vi "Send Update Data Buffer.vi"(6 "gain":dbl, 7 "Message Priority (Normal)":T2=enum."Normal", 8 "error in (no error)":errorcluster, 9 "dt":dbl, 10 "Data Buffer":T1, 11 "Message Enqueuer":refnum<class "Message Enqueuer.lvclass">) -> (0 "error out":errorcluster, 3 "Message Enqueuer out":refnum<class "Message Enqueuer.lvclass">)   [LabVIEW 2020, in "Calculation Worker.lvlib" / "Update Data Buffer Msg.lvclass"]
doc: "This VI sends the message to an actor."
uses:
  Update Data Buffer Msg.lvclass
  <vilib>/ActorFramework/Message Enqueuer/Message Enqueuer.lvclass
  <vilib>/ActorFramework/Message Enqueuer/Message Priority.ctl
  GPU FFT Calculator/GPU FFT Calculator/Data Source Buffer.ctl
  C:/Program Files/National Instruments/LabVIEW 2026/vi.lib/ActorFramework/Message/Message.lvclass
  Update Data Buffer Msg.lvclass/Update Data Buffer Msg.ctl
  <vilib>/ActorFramework/Message Enqueuer/Message Enqueuer.lvclass/Message Enqueuer.ctl
  <vilib>/ActorFramework/Message Priority Queue/Priority Enqueue.vi
  Data Source/Data Source/Data Source.lvclass
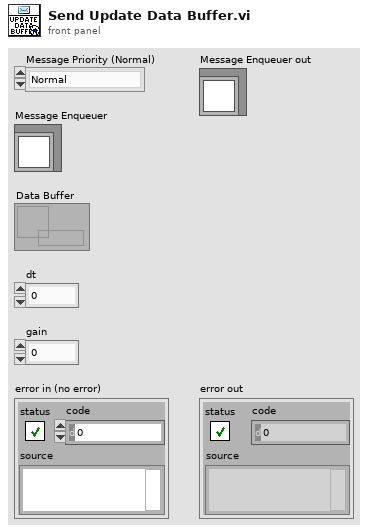
[diagram p1: front panel]
types:
  T1 = typedef "Data Source.lvlib/Data Source.lvclass/Data Source Buffer.ctl" = refnum<data-value>
  T2 = typedef "Actor Framework.lvlib/Message Enqueuer.lvclass/Message Priority.ctl" = enum16{"Low", "Normal", "High"}
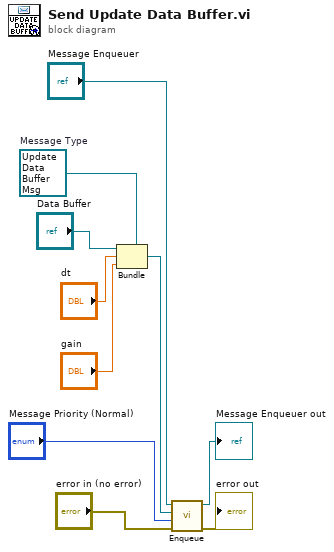
[diagram p0: block diagram]
diagram:
  w4 = refnum<class "Update Data Buffer Msg.lvclass"> refnum  # Message Type
  n1 = Bundle(cluster=w4, "Data Buffer", "dt", "gain") -> (w5:refnum<class "Update Data Buffer Msg.lvclass">)
  n2 = call <vilib>:"Enqueue.vi"("error in (no error)"="error in (no error)", "Message Priority (Normal)"="Message Priority (Normal)", "Message"=w5, "Message Enqueuer in"="Message Enqueuer") -> ("error out"=→"error out":errorcluster, "Message Enqueuer out"=→"Message Enqueuer out":refnum<class "Message Enqueuer.lvclass">)  [unwired: 6 in]
